vi "My_Server.vi"() -> ()   [LabVIEW 2019]
uses:
  <vilib>/G Open Source Project for LabVIEW/MQTT Broker/Server class/Server.lvclass/Server.ctl
  <vilib>/LabVIEW Open Source Project/MQTT TCP Connection/MQTT_TCP/Connection/TCPConnection.lvclass
  C:/Program Files (x86)/National Instruments/LabVIEW 2019/vi.lib/LabVIEW Open Source Project/MQTT Connection/MQTT_Connection/Connection/Connection.lvclass
  <vilib>/G Open Source Project for LabVIEW/MQTT Broker/Server class/Server.lvclass
  C:/Program Files (x86)/National Instruments/LabVIEW 2019/vi.lib/LabVIEW Open Source Project/MQTT Connection/MQTT_Base/Base Class/MQTT_Base.lvclass
  <vilib>/LabVIEW Open Source Project/MQTT Connection/MQTT_Base/Base Class/MQTT_Base.lvclass
  <vilib>/LabVIEW Open Source Project/MQTT Connection/MQTT_Connection/Connection/Connection.lvclass
panel:
  out "NbConnections":u32
  out "error server":errorcluster
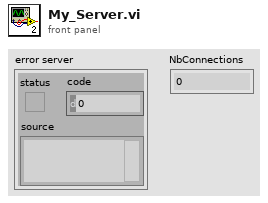
[diagram p1: front panel]
types:
  T1 = typedef "MQTT Server.lvlib/Server.lvclass/Public Events -- cluster.ctl" = cluster{"NbConnections":refnum<user-event>}
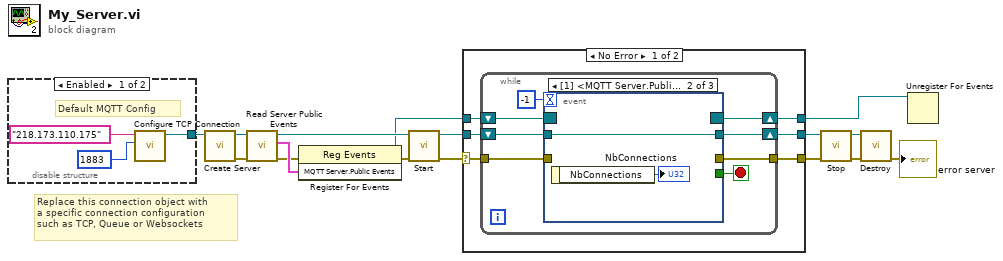
[diagram p0: block diagram]
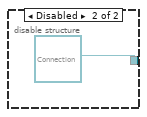
[diagram p2: hidden frame]
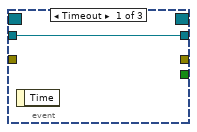
[diagram p3: hidden frame]
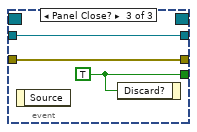
[diagram p4: hidden frame]
diagram:
  # "Replace this connection object with\na specific connection configuration\nsuch as TCP, Queue or Websockets"
  n1 = disable-structure shown="Enabled" {
    disable-tunnel: [w18 refnum<class "Connection.lvclass"> refnum ("Connection Configuration")] -> w16
    frame Enabled {
      # "Default MQTT Config"
      n2 = call <vilib>:"Configure TCP Connection.vi"("remote port (80)"=u16 1883, "address (localhost)"="218.173.110.175") -> ("TCPConnection"=w18:refnum<class "TCPConnection.lvclass">)  [unwired: 8 in, 1 out]
    }
    frame Disabled {
    }
  }
  n3 = call <vilib>:"Create Server.vi"("Connection Configuration"=w16) -> ("error out"=w2:errorcluster, "Server"=w1:refnum<class "Server.lvclass">)  [unwired: 9 in]
  n4 = call <vilib>:"Read Server Public Events.vi"("error in (no error)"=w2, "Server in"=w1) -> ("error out"=w3:errorcluster, "MQTT Server.Public Events"=w4:T1, "Server out"=w7:refnum<class "Server.lvclass">)  [unwired: 7 in]
  n5 = register-events(error in=w3, w4) -> (reference out=w5:refnum<event-registration>, error out=w9:errorcluster)  [unwired: 1 in]
  n6 = call <vilib>:"Start.vi"("error in (no error)"=w9, "MQTT_Base in"=w7) -> ("error out"=w10:errorcluster, "MQTT_Base out"=w8:refnum<class "Server.lvclass">)  [unwired: 7 in, 1 out]
  n7 = case shown="No Error" w10 {
    selector: w10 -> [w21 w41]
    tunnel: w8 -> [w26 w43]
    tunnel: [w25 w43] -> w13
    tunnel: w5 -> [w24 w42]
    tunnel: [w23 w42] -> w6
    tunnel: [w22 w41] -> w15
    frame No Error {
      n8 = while {
        shift-right: [w31] -> w25
        shift-left: w26 -> [w33]
        tunnel: [w28] -> w22
        tunnel: w21 -> [w27]
        shift-right: [w29] -> w23
        shift-left: w24 -> [w30]
        stop <- w32 stop-if-true
        n9 = event shown="[1] <MQTT Server.Public Events.NbConnections>: User Event" {
          selector: w30 -> [_ _ _]
          dyn-events: [_ _ _] -> w29
          timeout: -1 -> [_ _ _]
          tunnel: w33 -> [w35 w37 w40]
          tunnel: [_ _ w38] -> w32
          tunnel: [w35 w37 w40] -> w31
          tunnel: [_ _ w39] -> w28
          tunnel: w27 -> [_ _ w39]
          event Timeout {
            n10 = event-data() -> ()  [unwired: 1 in, 1 out]
          }
          event User Event {
            n11 = event-data() -> ("NbConnections"=→"NbConnections":u32)  [unwired: 1 in]
          }
          event Panel Close? {
            w38 = TRUE ("Discard?")
            n12 = event-data() -> ()  [unwired: 1 in, 1 out]
            n13 = event-data("Discard?"=w38) -> ()  [unwired: 1 in, 1 out]
          }
        }
      }
    }
    frame Error {
    }
  }
  n14 = call <vilib>:"Stop.vi"("error in (no error)"=w15, "MQTT_Base in"=w13) -> ("error out"=w14:errorcluster, "MQTT_Base out"=w12:refnum<class "Server.lvclass">)  [unwired: 7 in, 1 out]
  n15 = call <vilib>:"Destroy.vi"("error in (no error)"=w14, "MQTT_Base in"=w12) -> ("error out"=→"error server":errorcluster)  [unwired: 8 in, 1 out]
  n16 = Unregister For Events(event registration refnum=w6) -> ()  [unwired: 1 in, 1 out]
